vi "Interp_2D_Scattered_Data_2_Uniform.vi"(0 "X":dbl[](array[numeric])=[107.497559, 107.497559], 1 "method":i32(ring)=3 items=["nearest", "linear", "cubic", "biharmonic spline "], 2 "Interpolation Factor":i32=1, 5 "Y":dbl[](array[numeric])=[107.497559, 107.497559], 9 "U":dbl[](array[numeric])=[0.520245, 0.495578967376715], 11 "V":dbl[](array[numeric])=[1.605393, 2.2988169814147352]) -> (3 "IJ Values":i32[](array[numeric])=[1, 1], 4 "Xi":dbl[](array[numeric]), 6 "Yi":dbl[](array[numeric]), 8 "Ui":dbl[](array[numeric]), 10 "Vi":dbl[](array[numeric]), 15 "Convex Hull Check":dbl[](array[numeric]))   [LabVIEW 2011]
uses:
  <vilib>/Analysis/1siggen.llb/Ramp Pattern by Samples.vi
  <vilib>/gmath/interp.llb/Create Mesh Grid (2D) (x,y arrays).vi
  <vilib>/gmath/interp.llb/Interpolate 2D Scattered (2D).vi
  <vilib>/gmath/NI_Gmath.lvlib
  <vilib>/Analysis/NI_AALBase.lvlib
  <vilib>/gmath/NI_AAL_Interpolation.lvlib
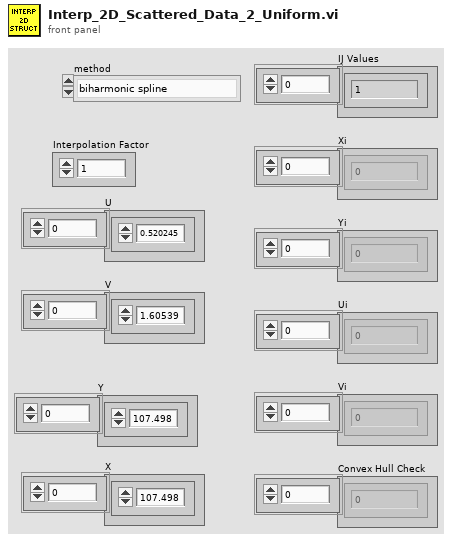
[diagram p1: front panel]
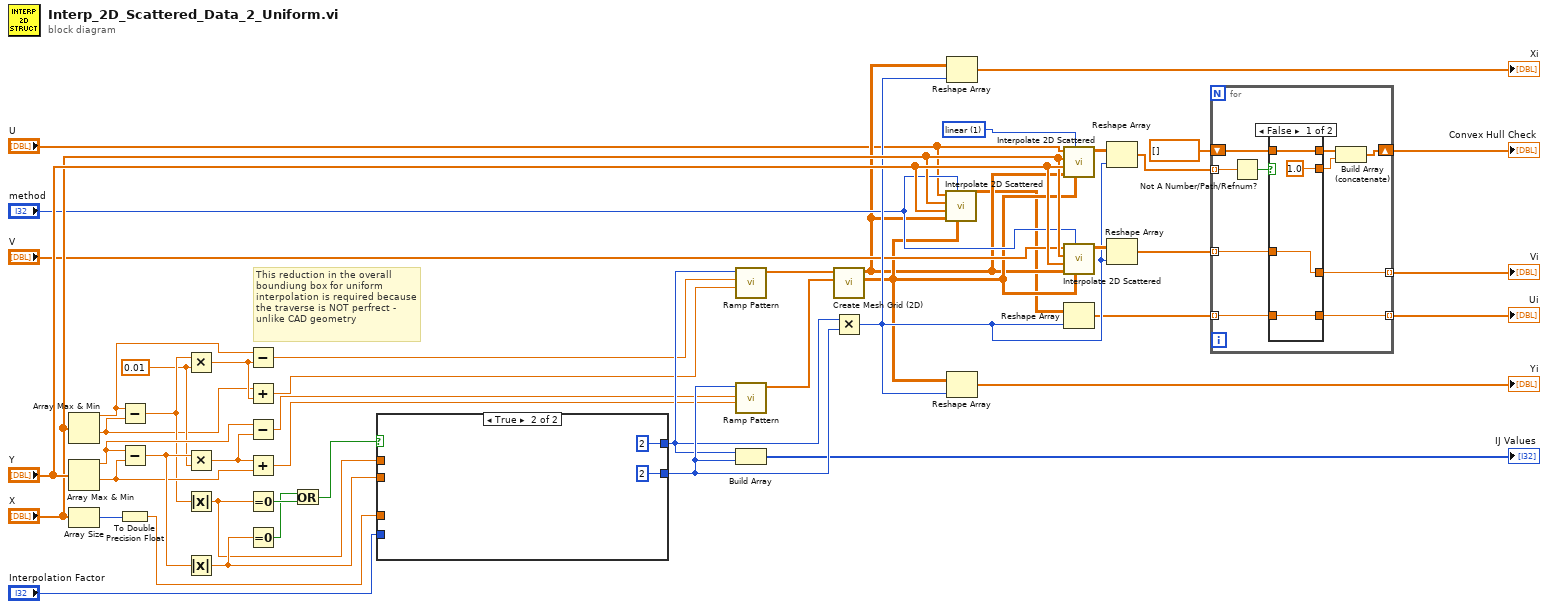
[diagram p0: block diagram]
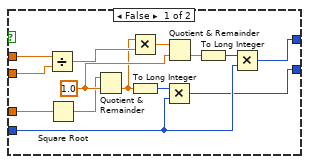
[diagram p2: hidden frame]
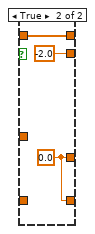
[diagram p3: hidden frame]
diagram:
  w6 = 0.01 ("y")
  w40 = 1 items=["nearest", "linear", "cubic", "biharmonic spline "] ("method")
  # "This reduction in the overall boundiung box for uniform interpolation is required because the traverse is NOT perfrect - unlike CAD geometry"
  n1 = Array Max & Min(array="X") -> (max value=w2:dbl, min value=w4:dbl)  [unwired: 2 out]
  n2 = Array Max & Min(array="Y") -> (max value=w10:dbl, min value=w12:dbl)  [unwired: 2 out]
  n3 = Array Size(array="X") -> (size(s)=w42:i32)
  n4 = Subtract(x=w2, y=w4) -> (x-y=w7:dbl)
  n5 = Subtract(x=w10, y=w12) -> (x-y=w14:dbl)
  n6 = To Double Precision Float(number=w42) -> (double precision float=w43:dbl)
  n7 = Multiply(x=w7, y=w6) -> (x*y=w5:dbl)
  n8 = Multiply(x=w14, y=w6) -> (x*y=w13:dbl)
  n9 = Absolute Value(x=w7) -> (abs(x)=w23:dbl)
  n10 = Absolute Value(x=w14) -> (abs(x)=w24:dbl)
  n11 = Subtract(x=w2, y=w5) -> (x-y=w1:dbl)
  n12 = Add(x=w4, y=w5) -> (x+y=w3:dbl)
  n13 = Subtract(x=w10, y=w13) -> (x-y=w9:dbl)
  n14 = Add(x=w13, y=w12) -> (x+y=w11:dbl)
  n15 = Equal To 0?(x=w23) -> (x = 0?=w22:bool)
  n16 = Equal To 0?(x=w24) -> (x = 0?=w21:bool)
  n17 = Or(x=w21, y=w22) -> (x .or. y?=w8:bool)
  n18 = case shown="True" w8 {
    tunnel: "Interpolation Factor" -> [w61 _]
    tunnel: [w59 2] -> w45
    tunnel: [w57 2] -> w44
    tunnel: w23 -> [w54 _]
    tunnel: w43 -> [w50 _]
    tunnel: w24 -> [w48 _]
    frame False {
      w55 = 1.0 ("y")
      n19 = Divide(x=w54, y=w48) -> (x/y=w53:dbl)
      n20 = Square Root(x=w50) -> (sqrt(x)=w51:dbl)
      n21 = Quotient & Remainder(x=w51, y=w55) -> (floor(x/y)=w52:dbl)  [unwired: 1 out]
      n22 = Multiply(x=w52, y=w53) -> (x*y=w49:dbl)
      n23 = To Long Integer(number=w52) -> (32bit integer=w60:i32)
      n24 = Multiply(x=w60, y=w61) -> (x*y=w59:i32)
      n25 = Quotient & Remainder(x=w49, y=w55) -> (floor(x/y)=w56:dbl)  [unwired: 1 out]
      n26 = To Long Integer(number=w56) -> (32bit integer=w58:i32)
      n27 = Multiply(x=w58, y=w61) -> (x*y=w57:i32)
    }
    frame True {
    }
  }
  n28 = call-poly <vilib>:"Ramp Pattern.vi"("start"=w3, "end"=w1, "samples"=w44) -> ("Ramp Pattern"=w18:dbl[])  [unwired: 7 in, 1 out]
  n29 = call-poly <vilib>:"Ramp Pattern.vi"("start"=w11, "end"=w9, "samples"=w45) -> ("Ramp Pattern"=w19:dbl[])  [unwired: 7 in, 1 out]
  n30 = Build Array(w44, w45) -> (→"IJ Values":i32[])
  n31 = call-poly <vilib>:"Create Mesh Grid (2D).vi"("y domain"=w19, "x domain"=w18) -> ("Y"=w20:dbl[][], "X"=w17:dbl[][])  [unwired: 7 in, 1 out]
  n32 = Multiply(x=w44, y=w45) -> (x*y=w36:i32)
  n33 = call-poly <vilib>:"Interpolate 2D Scattered.vi"("Yi"=w20, "method"="method", "Xi"=w17, "Y"="Y", "X"="X", "Z"="U") -> ("Zi"=w15:dbl[][])  [unwired: 4 in, 1 out]
  n34 = Reshape Array(w17, w36) -> (→"Xi":dbl[])
  n35 = Reshape Array(w20, w36) -> (→"Yi":dbl[])
  n36 = call-poly <vilib>:"Interpolate 2D Scattered.vi"("Yi"=w20, "method"=w40, "Xi"=w17, "Y"="Y", "X"="X", "Z"="U") -> ("Zi"=w28:dbl[][])  [unwired: 4 in, 1 out]
  n37 = call-poly <vilib>:"Interpolate 2D Scattered.vi"("Yi"=w20, "method"="method", "Xi"=w17, "Y"="Y", "X"="X", "Z"="V") -> ("Zi"=w39:dbl[][])  [unwired: 4 in, 1 out]
  n38 = Reshape Array(w15, w36) -> (w32:dbl[])
  n39 = Reshape Array(w28, w36) -> (w29:dbl[])
  n40 = Reshape Array(w39, w36) -> (w33:dbl[])
  n41 = for {
    shift-right: [w73] -> w30
    shift-left: dbl[] [] ("output array") -> [w71]
    tunnel: w29 -> [w65] mode=indexing
    tunnel: w32 -> [w66] mode=indexing
    tunnel: w33 -> [w69] mode=indexing
    tunnel: [w68] -> w34 mode=indexing
    tunnel: [w67] -> w35 mode=indexing
    n42 = Not A Number/Path/Refnum?(number/path/refnum=w65) -> (NaN/Path/Refnum?=w64:bool)
    n43 = case shown="False" w64 {
      tunnel: [w77 w80] -> w72
      tunnel: w71 -> [w77 w80]
      tunnel: [1.0 -2.0] -> w70
      tunnel: w66 -> [w75 _]
      tunnel: w69 -> [w74 _]
      tunnel: [w75 w78] -> w68
      tunnel: [w74 w78] -> w67
      frame False {
      }
      frame True {
        w78 = 0.0
      }
    }
    n44 = Build Array (concatenate)(w72, w70) -> (w73:dbl[])
  }
  "Vi" <- w35
  "Ui" <- w34
  "Convex Hull Check" <- w30
